vi "Create Cell.vi"(5 "Cell Generic Format":T1={"Format Cell Cluster"={"Font Ref"=refnum, "Leading"=18.0, "Horizontal Aligment"=enum."JUSTIFY", "Vertical Alignment"=enum."BOTTOM"}, "Line"={"Thickness"=0.5, "Color"=0}, "Borders and BG"={"Cell Border"=0, "BG"=16777225}, "PdfPCell refnum"=refnum}, 11 "error in (no error)":errorcluster) -> (6 "PdfP Cell ref":refnum<k24>, 8 "Font Ref":refnum<k24>, 15 "error out":errorcluster)   [LabVIEW 2013]
doc: "Version 1.0\nDeveloped by Jean-Marc Simard\nCopyright © 2010, Exaprom Inc.\nAll rights reserved.\nLicense: BSD\n\nWith iTextSharp 4.1.6 (http://itextsharp.sourceforge.net)\nunder Mozilla Public License Version 1.1\n(http://www.mozilla.org/MPL/MPL-1.1.html)"
uses:
  C:/Users/MaxCorp/Documents/GitHub/TopView/DLL/itextsharp.dll
  DLL/itextsharp.dll
  Controls/Cell Generic Format with FOnt refnum.ctl
  Controls/Cell Cluster.ctl
  Controls/Font size.ctl
  Controls/Texte alignement.ctl
  Controls/Cell Vertical alignment.ctl
  Controls/Cell Border.ctl
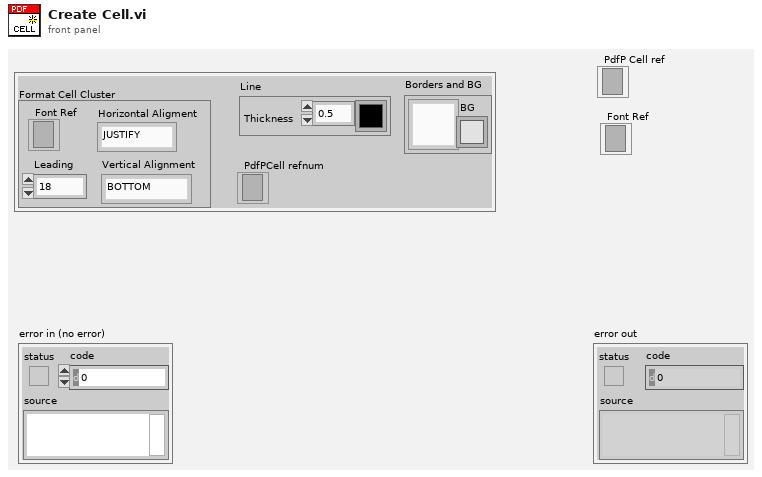
[diagram p1: front panel]
types:
  T1 = typedef "Cell Generic Format with FOnt refnum.ctl" = cluster{"Format Cell Cluster":T2, "Line":cluster{"Thickness":sgl, "Color":u32}, "Borders and BG":cluster{"Cell Border":T6, "BG":u32}, "PdfPCell refnum":refnum<k24>}
  T2 = typedef "Cell Cluster.ctl" = cluster{"Font Ref":refnum<k24>, "Leading":T3, "Horizontal Aligment":T4, "Vertical Alignment":T5}
  T3 = typedef "Font size.ctl" = sgl
  T4 = typedef "Texte alignement.ctl" = enum16{"Select", "CENTER", "JUSTIFY", "LEFT", "RIGHT"}
  T5 = typedef "Cell Vertical alignment.ctl" = enum16{"TOP", "MIDDLE", "BOTTOM"}
  T6 = typedef "Cell Border.ctl" = u16
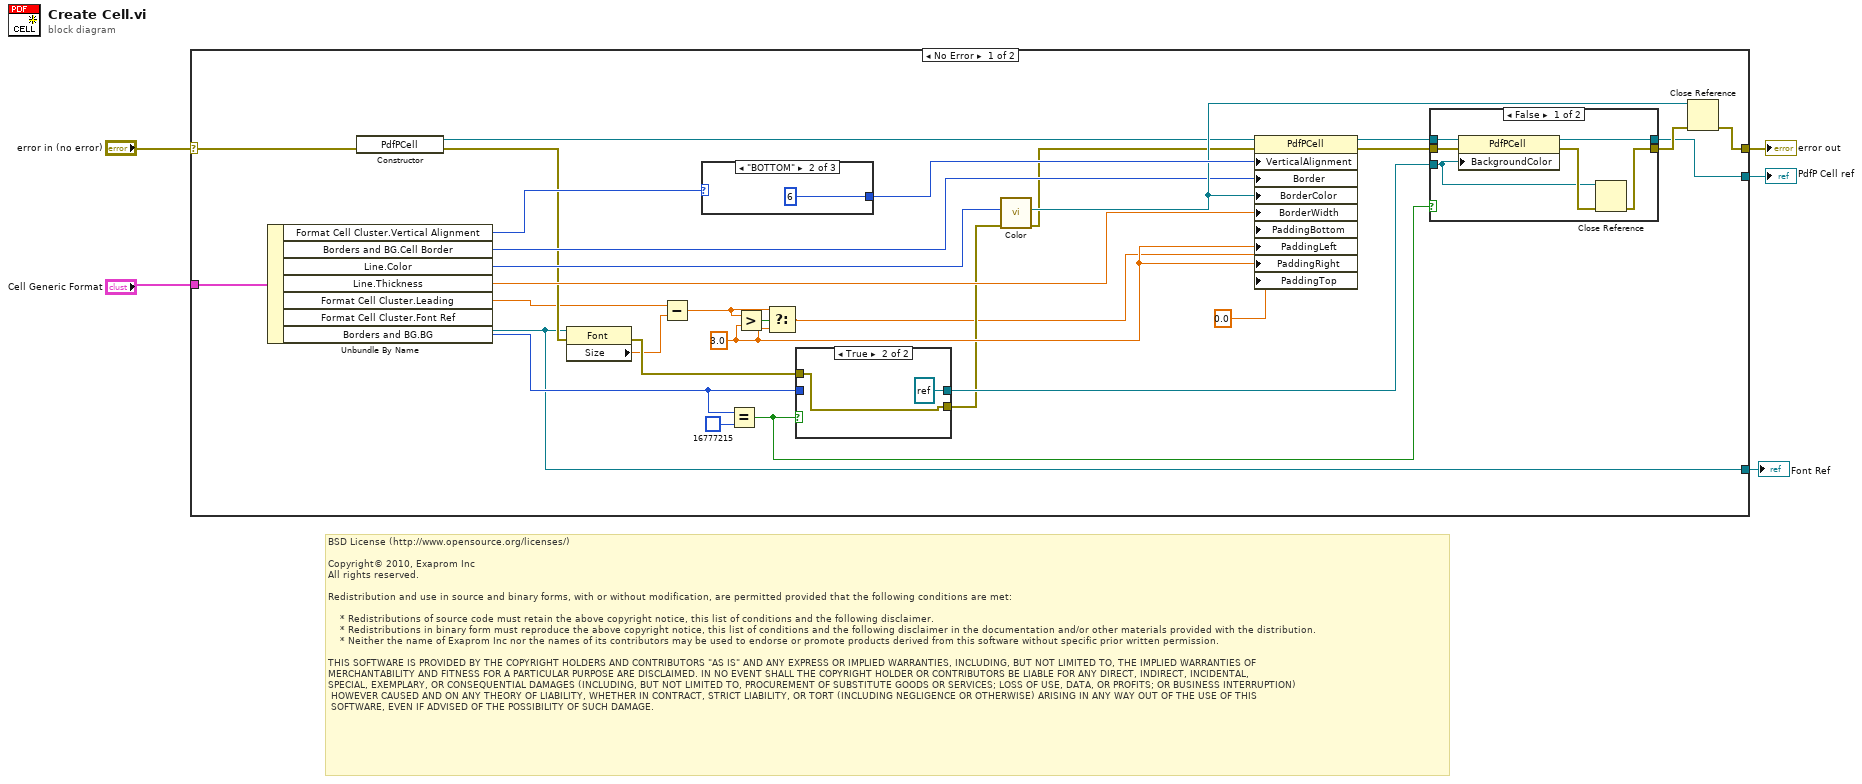
[diagram p0: block diagram]
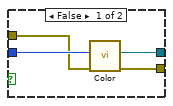
[diagram p2: hidden frame]
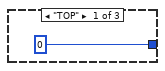
[diagram p4: hidden frame]
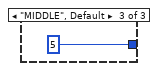
[diagram p5: hidden frame]
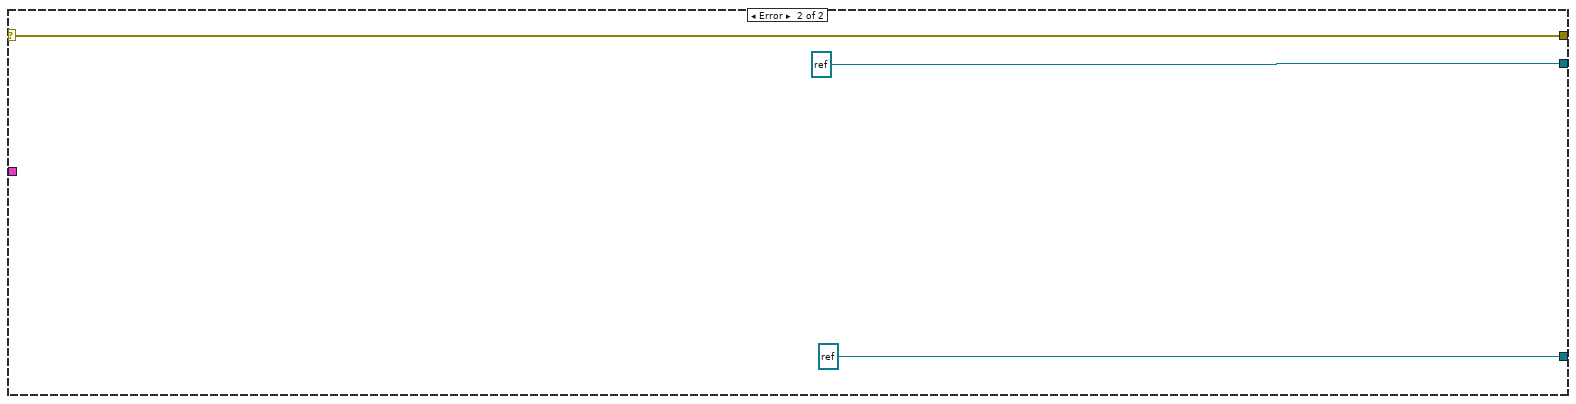
[diagram p6: hidden frame]
diagram:
  # "BSD License (http://www.opensource.org/licenses/)\n\nCopyright© 2010, Exaprom Inc\nAll rights reserved.\n\nRedistribution and use in source and binary forms, with or without modification, are permitted provided that the following conditions are met:\n\n    * Redistributions of source code must retain the above copyright notice, this list of conditions and the following disclaimer.\n    * Redistributions in binary form must reproduce the above copyright notice, this list of conditions and the following disclaimer in the documentation and/or other materials provided with the distribution.\n    * Neither the name of Exaprom Inc nor the names of its contributors may be used to endorse or promote products derived from this software without specific prior written permission.\n\nTHIS SOFTWARE IS PROVIDED BY THE COPYRIGHT HOLDERS AND CONTRIBUTORS \"AS IS\" AND ANY EXPRESS OR IMPLIED WARRANTIES, INCLUDING, BUT NOT LIMITED TO, THE IMPLIED WARRANTIES OF \nMERCHANTABILITY AND FITNESS FOR A PARTICULAR PURPOSE ARE DISCLAIMED. IN NO EVENT SHALL THE COPYRIGHT HOLDER OR CONTRIBUTORS BE LIABLE FOR ANY DIRECT, INDIRECT, INCIDENTAL,\nSPECIAL, EXEMPLARY, OR CONSEQUENTIAL DAMAGES (INCLUDING, BUT NOT LIMITED TO, PROCUREMENT OF SUBSTITUTE GOODS OR SERVICES; LOSS OF USE, DATA, OR PROFITS; OR BUSINESS INTERRUPTION)\n HOWEVER CAUSED AND ON ANY THEORY OF LIABILITY, WHETHER IN CONTRACT, STRICT LIABILITY, OR TORT (INCLUDING NEGLIGENCE OR OTHERWISE) ARISING IN ANY WAY OUT OF THE USE OF THIS\n SOFTWARE, EVEN IF ADVISED OF THE POSSIBILITY OF SUCH DAMAGE."
  n1 = case shown="No Error" "error in (no error)" {
    selector: "error in (no error)" -> [w35 w55]
    tunnel: [w21 w55] -> w4
    tunnel: [w22 refnum<k24> refnum ("new reference")] -> w3
    tunnel: "Cell Generic Format" -> [w30 _]
    tunnel: [w8 refnum<k24> refnum ("Font Ref")] -> w1
    frame No Error {
      w31 = sgl 3.0 ("t")
      n2 = Unbundle By Name(w30) -> ("Format Cell Cluster.Vertical Alignment"=w20:T5, "Borders and BG.Cell Border"=w19:T6, "Line.Color"=w18:u32, "Line.Thickness"=w17:sgl, "Format Cell Cluster.Leading"=w10:T3, "Format Cell Cluster.Font Ref"=w8:refnum<k24>, "Borders and BG.BG"=w16:u32)
      n3 = constructor class="PdfPCell"(error in=w35) -> (reference out=w23:refnum<k24>, error out=w13:errorcluster)  [unwired: 2 in, 1 out]
      n4 = property class="Font"(reference=w8, error in=w13) -> (error out=w15:errorcluster, "Size"=w9:sgl)  [unwired: 1 out]
      n5 = Subtract(x=w10, y=w9) -> (x-y=w32:T3)
      n6 = case shown="\"BOTTOM\"" w20 {
        tunnel: [0 6 5] -> w34
        frame "TOP" {
        }
        frame "BOTTOM" {
        }
        frame "MIDDLE", Default {
        }
      }
      n7 = Equal?(x=w16, y=u32 16777215 ("Color")) -> (x = y?=w11:bool)
      n8 = Greater?(x=w32, y=w31) -> (0:w33:bool)
      n9 = Select(t=w32, s=w33, f=w31) -> (s? t:f=w7:T3)
      n10 = case shown="True" w11 {
        tunnel: [w39 refnum<k24> refnum ("Color")] -> w24
        tunnel: w16 -> [w38 _]
        tunnel: w15 -> [w37 w40]
        tunnel: [w36 w40] -> w14
        frame False {
          n11 = call "Color.vi"("error in (no error)"=w37, "Color"=w38) -> ("error out"=w36:errorcluster, "Color"=w39:refnum<k24>)  [unwired: 8 out]
        }
        frame True {
        }
      }
      n12 = call "Color.vi"("error in (no error)"=w14, "Color"=w18) -> ("error out"=w12:errorcluster, "Color"=w25:refnum<k24>)  [unwired: 8 out]
      n13 = property class="PdfPCell"(reference=w23, error in=w12, "VerticalAlignment"=w34, "Border"=w19, "BorderColor"=w25, "BorderWidth"=w17, "PaddingBottom"=w7, "PaddingLeft"=w31, "PaddingRight"=w31, "PaddingTop"=sgl 0.0) -> (reference out=w26:refnum<k24>, error out=w29:errorcluster)
      n14 = case shown="False" w11 {
        tunnel: w26 -> [w47 w49]
        tunnel: w29 -> [w46 w48]
        tunnel: [w45 w49] -> w22
        tunnel: [w44 w48] -> w28
        tunnel: w24 -> [w42 _]
        frame False {
          n15 = property class="PdfPCell"(reference=w47, error in=w46, "BackgroundColor"=w42) -> (reference out=w45:refnum<k24>, error out=w43:errorcluster)
          n16 = Close Reference(reference=w42, error in (no error)=w43) -> (error out=w44:errorcluster)
        }
        frame True {
        }
      }
      n17 = Close Reference(reference=w25, error in (no error)=w28) -> (error out=w21:errorcluster)
    }
    frame Error {
    }
  }
  "error out" <- w4
  "PdfP Cell ref" <- w3
  "Font Ref" <- w1
